vi "Call ReentrantVi.vi"(8 "error in (no error)":errorcluster caption="错误输入（无错误）", 10 "Vi Path":path, 11 "PanelDataNode 输入":refnum<class "PanelDataNode.lvclass"> caption="DNL_LabVIEW Object in") -> (0 "error out":errorcluster caption="错误输出", 2 "VI*":refnum<vi>, 3 "PanelDataNode 输出":refnum<class "PanelDataNode.lvclass"> caption="DNL_LabVIEW Object out")   [LabVIEW 2016, in "PanelDataNode.lvclass"]
uses:
  PanelDataNode.lvclass
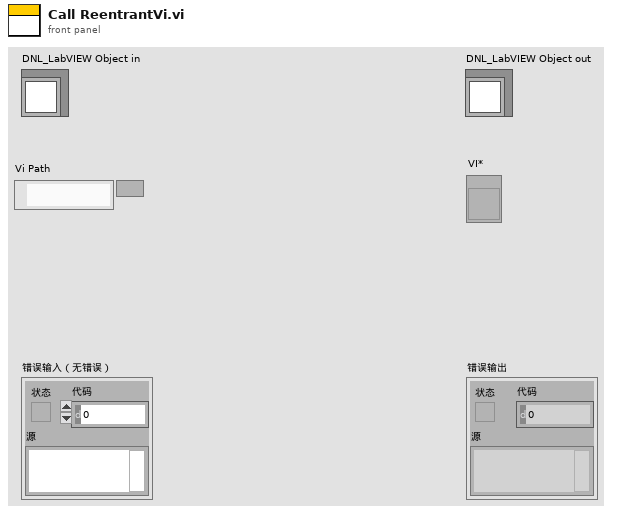
[diagram p1: front panel]
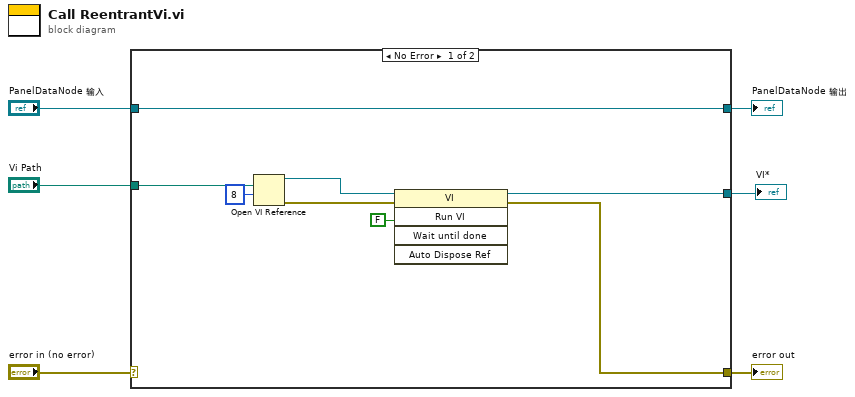
[diagram p0: block diagram]
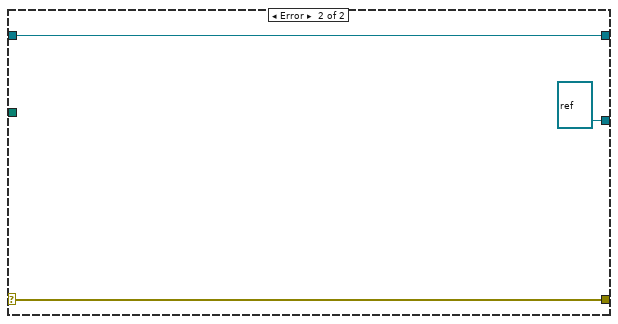
[diagram p2: hidden frame]
diagram:
  n1 = case shown="No Error" "error in (no error)" {
    selector: "error in (no error)" -> [_ w17]
    tunnel: [w7 w17] -> w5
    tunnel: [w14 w16] -> w3
    tunnel: "PanelDataNode 输入" -> [w14 w16]
    tunnel: "Vi Path" -> [w13 _]
    tunnel: [w9 refnum<vi> refnum ("vi reference")] -> w1
    frame No Error {
      n2 = Open VI Reference(vi path=w13, options=8 ("选项")) -> (vi reference=w11:refnum<vi>, error out=w8:errorcluster)  [unwired: 4 in]
      n3 = invoke class="VI" method="Run VI"(reference=w11, error in=w8, "Wait until done"=FALSE ("结束前等待")) -> (reference out=w9:refnum<vi>, error out=w7:errorcluster)  [unwired: 2 in, 3 out]
    }
    frame Error {
    }
  }
  "error out" <- w5
  "PanelDataNode 输出" <- w3
  "VI*" <- w1
